vi "all-signals-expressvi.vi"() -> ()   [LabVIEW 2018]
uses:
  <vilib>/express/express shared/transition.llb/Dynamic To Waveform Array.vi
  <vilib>/express/express signal manip/GetorSetDDTAttributes/Set DDT Attributes/SetT0.vi
  <vilib>/express/express shared/transition.llb/Waveform Array To Dynamic.vi
  <vilib>/express/express signal manip/GetorSetDDTAttributes/Set DDT Attributes/Set DDT Properties.xnode
panel:
  in  "Clear Charts":bool
  in  "Messzeit in ms":u32=100 min=10 max=1000 step=10
  out "Bremsmoment":dynamicdata(graph)
  out "Strom, Spannung, elektrische Leistung":dynamicdata(graph)
  out "Geschwindigkeit":dynamicdata(graph)
  in  "stop (F)":bool
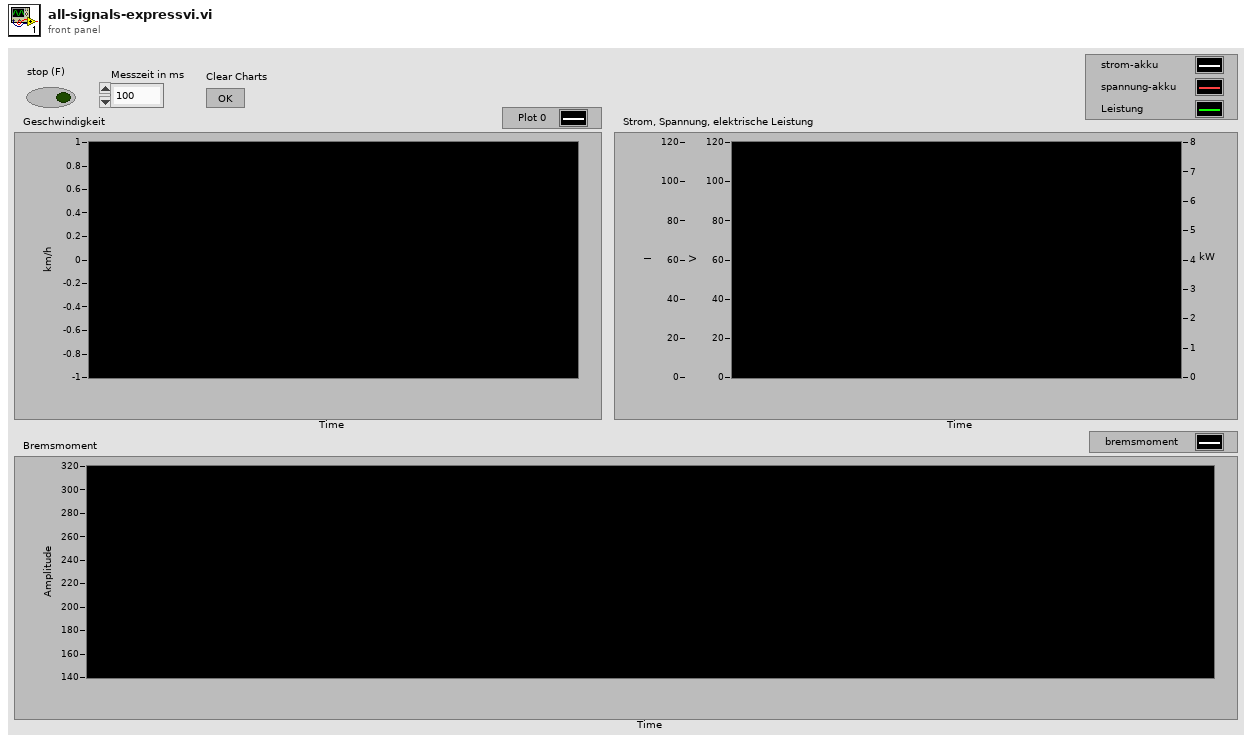
[diagram p1: front panel]
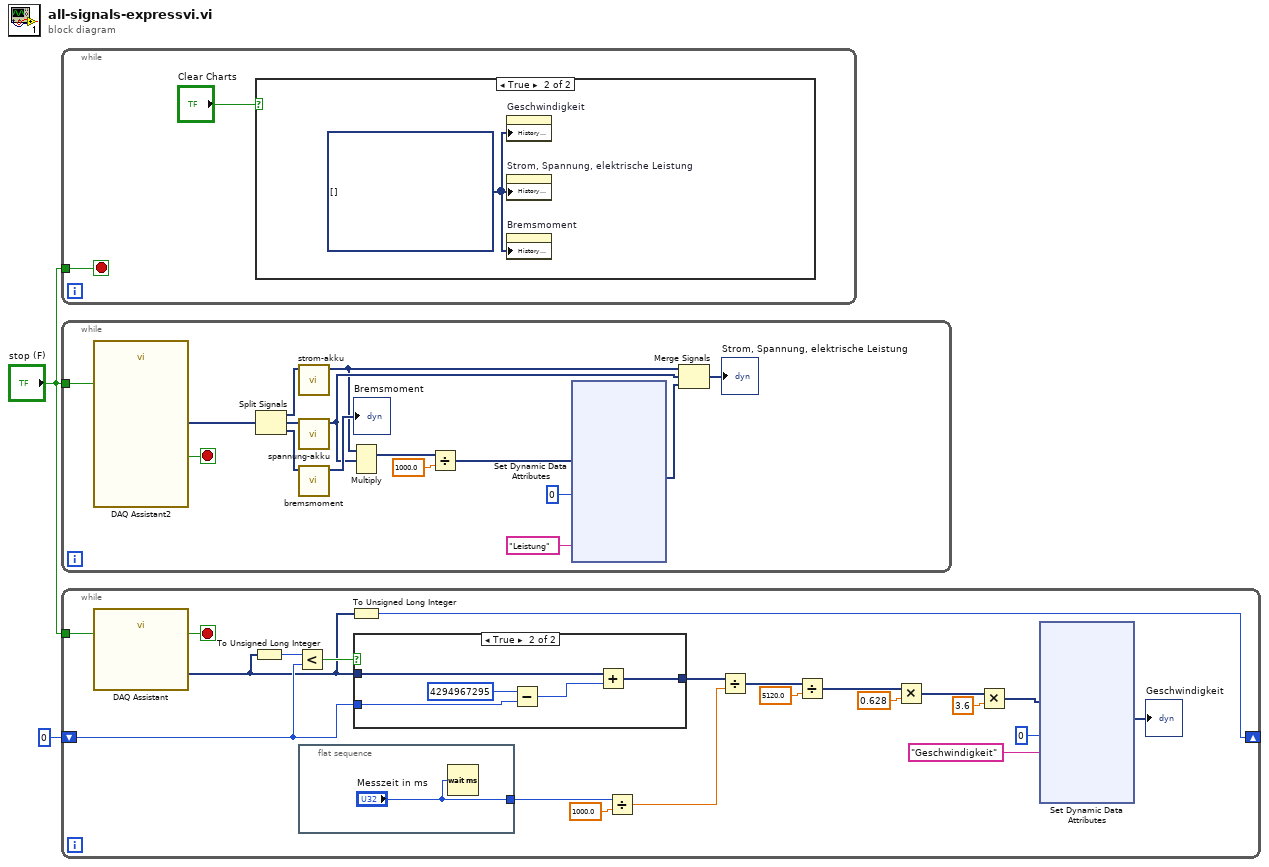
[diagram p0: block diagram]
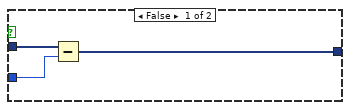
[diagram p3: hidden frame]
diagram:
  n1 = while {
    tunnel: "stop (F)" -> [w3]
    stop <- w3 stop-if-true
    n2 = case shown="True" "Clear Charts" {
      frame False {
      }
      frame True {
        w5 = dynamicdata[] [] ("History Data")
        n3 = property on="Geschwindigkeit" class="WFChart (strict)"("History Data"=w5) -> ()  [unwired: 2 in, 2 out]
        n4 = property on="Strom, Spannung, elektrische Leistung" class="WFChart (strict)"("History Data"=w5) -> ()  [unwired: 2 in, 2 out]
        n5 = property on="Bremsmoment" class="WFChart (strict)"("History Data"=w5) -> ()  [unwired: 2 in, 2 out]
      }
    }
  }
  n6 = while {
    tunnel: "stop (F)" -> [w14]
    stop <- w15 stop-if-true
    n7 = call "DAQ Assistant2"("stop (F)"=w14) -> ("data"=w16:dynamicdata, "stopped"=w15:bool)  [unwired: 15 in, 2 out]
    n8 = Split Signals(w16) -> (w21:dynamicdata, w20:dynamicdata, w19:dynamicdata)  [unwired: 3 in]
    n9 = call "strom-akku.vi"("Dynamic Data"=w21) -> ("Filtered Signal"=w12:dynamicdata)  [unwired: 10 in]
    n10 = call "spannung-akku.vi"("Dynamic Data in"=w20) -> ("Dynamic Data out"=w13:dynamicdata)  [unwired: 10 in]
    n11 = call "bremsmoment.vi"("Dynamic Data in"=w19) -> ("Dynamic Data out"=→"Bremsmoment":dynamicdata)  [unwired: 10 in]
    n12 = Multiply(1:w13, 2:w12) -> (0:w10:dynamicdata)  [unwired: 1 in, 1 out]
    n13 = Divide(x=w10, y=1000.0) -> (x/y=w9:dynamicdata)
    n14 = xnode "Set Dynamic Data Attributes"("Signals In"=w9, "Signal Index"=0, "Signal Name"="Leistung") -> ("Signals Out"=w8:dynamicdata)  [unwired: 1 in, 1 out]
    n15 = Merge Signals(w12, w13, w8) -> (→"Strom, Spannung, elektrische Leistung":dynamicdata)
  }
  n16 = while {
    shift-right: [w49] -> _
    shift-left: u32 0 -> [w48]
    tunnel: "stop (F)" -> [w45]
    stop <- w44 stop-if-true
    n17 = call "DAQ Assistant"("stop (F)"=w45) -> ("data"=w47:dynamicdata, "stopped"=w44:bool)  [unwired: 15 in, 2 out]
    n18 = To Unsigned Long Integer(number=w47) -> (unsigned 32bit integer=w46:u32)
    n19 = Less?(x=w46, y=w48) -> (x < y?=w55:bool)
    n20 = flat-sequence {
      tunnel: ["Messzeit in ms"] -> w43
      frame #0 {
        n21 = Wait (ms)(milliseconds to wait="Messzeit in ms") -> ()  [unwired: 1 out]
      }
    }
    n22 = To Unsigned Long Integer(number=w47) -> (unsigned 32bit integer=w49:u32)
    n23 = case shown="True" w55 {
      tunnel: w47 -> [w72 w74]
      tunnel: w48 -> [w71 w76]
      tunnel: [w70 w73] -> w41
      frame False {
        n24 = Subtract(x=w72, y=w71) -> (x-y=w70:dynamicdata)
      }
      frame True {
        n25 = Subtract(x=u32 4294967295, y=w76) -> (x-y=w75:u32)
        n26 = Add(x=w74, y=w75) -> (x+y=w73:dynamicdata)
      }
    }
    n27 = Divide(x=w43, y=1000.0) -> (x/y=w40:dbl)
    n28 = Divide(x=w41, y=w40) -> (x/y=w39:dynamicdata)
    n29 = Divide(x=w39, y=5120.0) -> (x/y=w53:dynamicdata)
    n30 = Multiply(x=w53, y=0.628) -> (x*y=w50:dynamicdata)
    n31 = Multiply(x=w50, y=3.6) -> (x*y=w36:dynamicdata)
    n32 = xnode "Set Dynamic Data Attributes"("Signals In"=w36, "Signal Index"=0, "Signal Name"="Geschwindigkeit") -> ("Signals Out"=→"Geschwindigkeit":dynamicdata)  [unwired: 1 in, 1 out]
  }
